vi "Revised-List_Extractor-Mar31.vi"(5 "Input Cluster":T2, 11 "error in (no error)":errorcluster) -> (6 "Output Cluster":T1, 15 "error out":errorcluster)   [LabVIEW 2014]
doc: "This VI extracts and arranges the list of species in an array.\nIn_Arr : Array of species to be arranged\nOut_Arr : Arranged array.\nNote: It does not process list of \"Kinetic Laws\" \n\nDesigned By:\nHB\nhaba@dtu.dk"
panel:
  out "Sp_for_ODE+Names":string[](array[string])
  out "SP_for_ODE_Init_Amnt":string[](array[string])
  out "Sp_for_ODE":string[](array[string])
  out "Ex_Mod_Init_Amnt":string[](array[string])
  out "Rest_Sp_IDs":string[](array[string])
  out "Rest_Sp_Init_Amnt":string[](array[string])
  out "Rest_Sp_IDs+Names":string[](array[string])
  out "Sp_Init_Amount":string[](array[string])
  out "All_Mods":string[](array[string])
  out "Products_Arr":string[](array[string])
  out "Reactants_Arr":string[](array[string])
  out "Ex_Mod_IDs":string[](array[string])
  out "Sp_ID":string[](array[string])
  out "Sp_Name":string[](array[string])
  out "Mod_In_Arr":string[](array[string])
  out "Ex_Mod_IDs+Names":string[](array[string])
  out "strng":string
  out "New mods":string[](array[string])
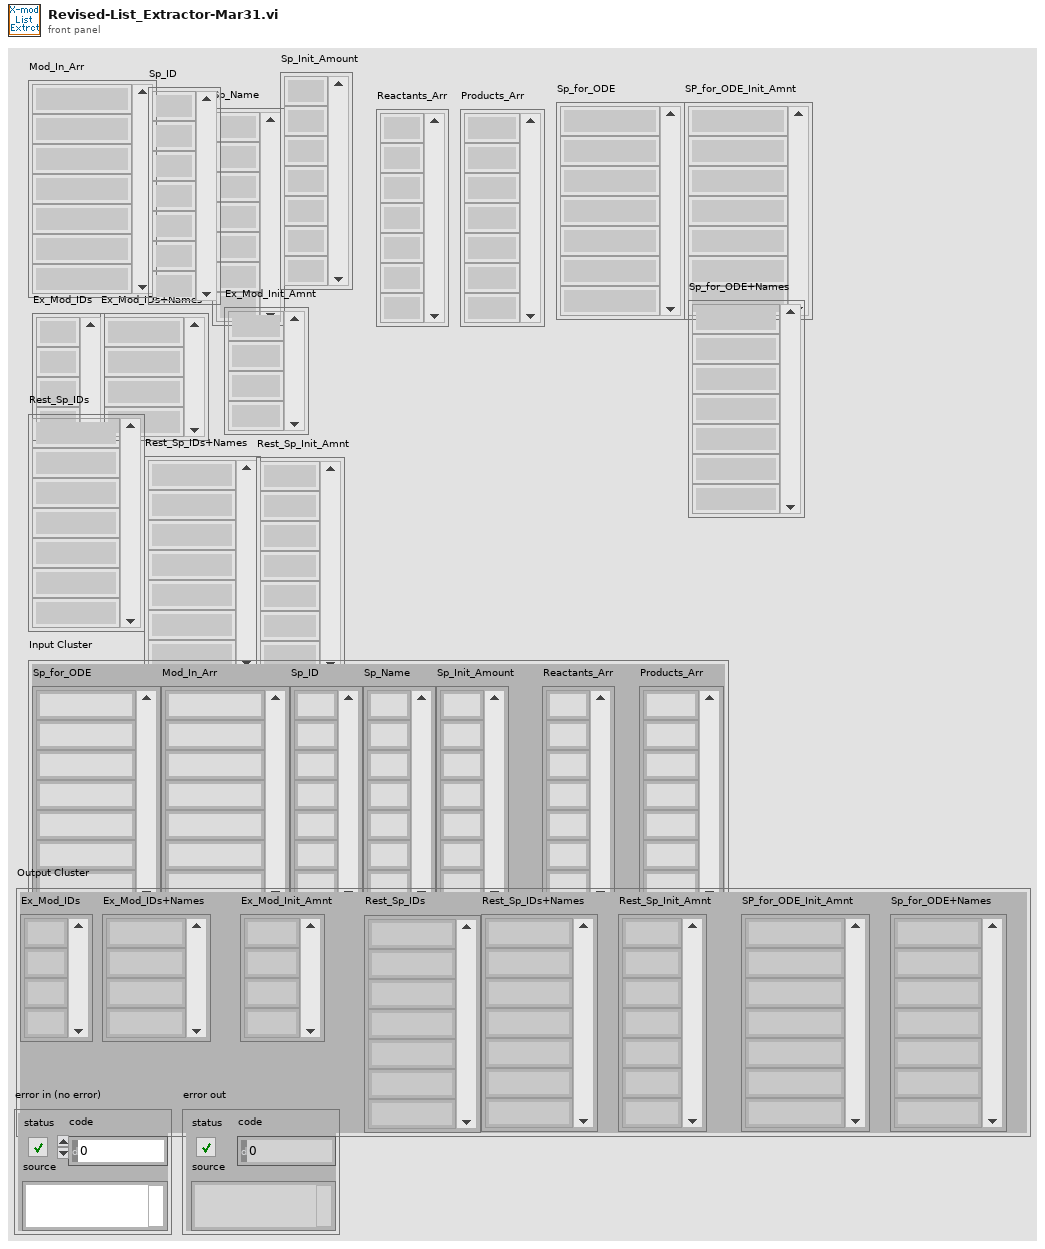
[diagram p1: front panel]
types:
  T1 = cluster{"Ex_Mod_IDs":string[], "Ex_Mod_IDs+Names":string[], "Ex_Mod_Init_Amnt":string[], "Rest_Sp_IDs ":string[], "Rest_Sp_IDs+Names":string[], "Rest_Sp_Init_Amnt":string[], "SP_for_ODE_Init_Amnt":string[], "Sp_for_ODE+Names":string[]}
  T2 = cluster{"Sp_for_ODE":string[], "Mod_In_Arr":string[], "Sp_ID ":string[], "Sp_Name":string[], "Sp_Init_Amount":string[], "Reactants_Arr ":string[], "Products_Arr":string[]}
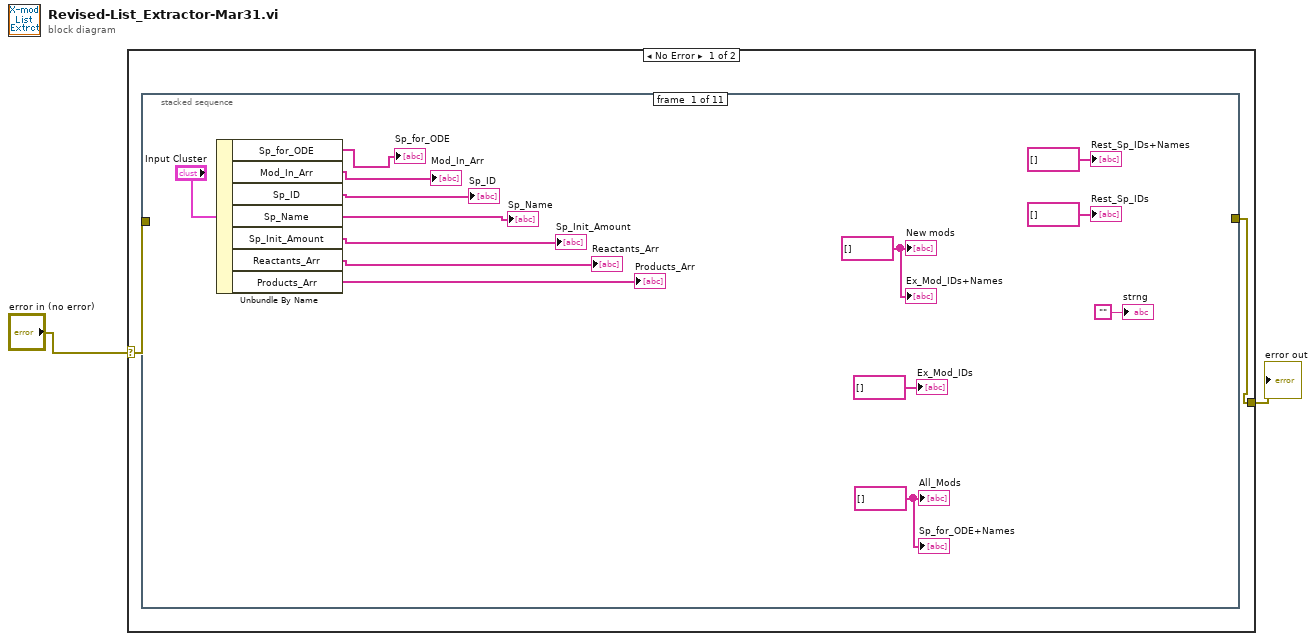
[diagram p0: block diagram]
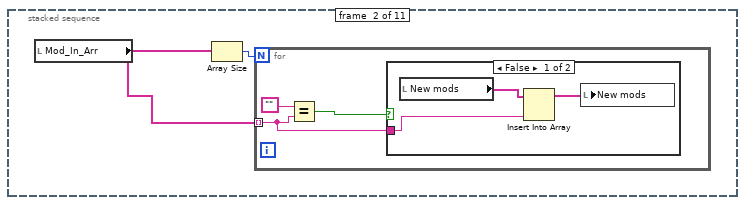
[diagram p2: hidden frame]
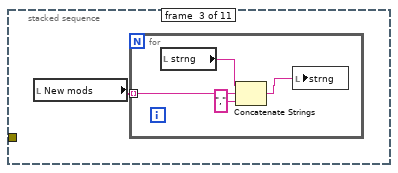
[diagram p4: hidden frame]
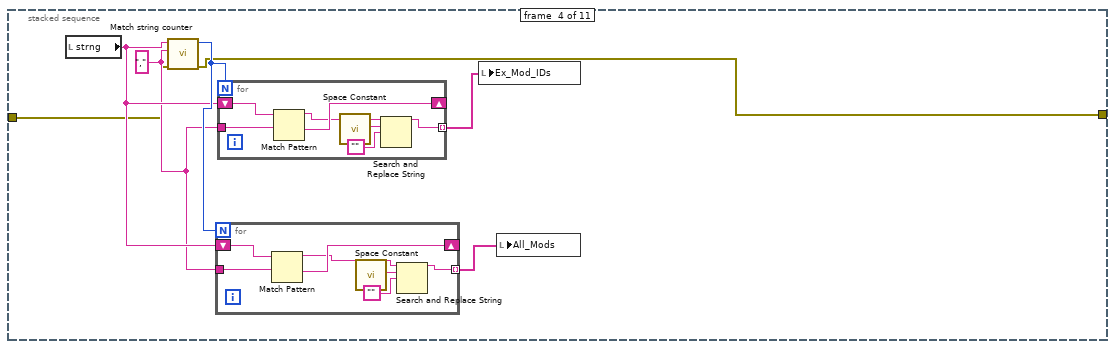
[diagram p5: hidden frame]
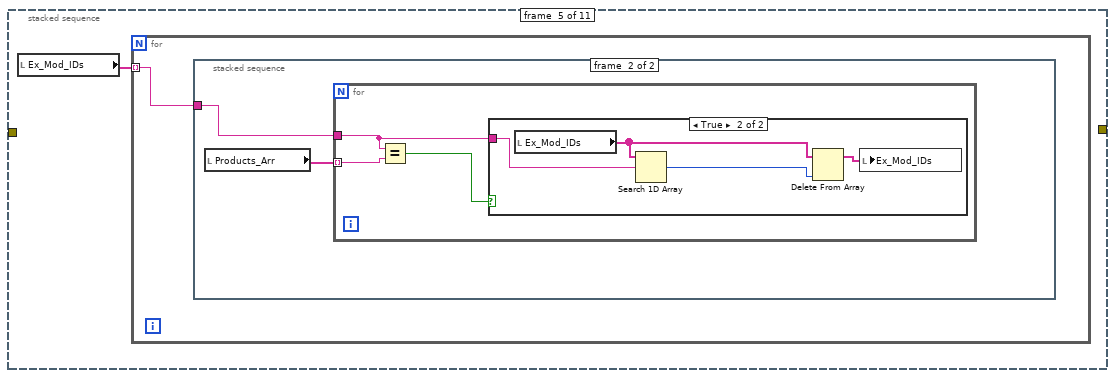
[diagram p6: hidden frame]
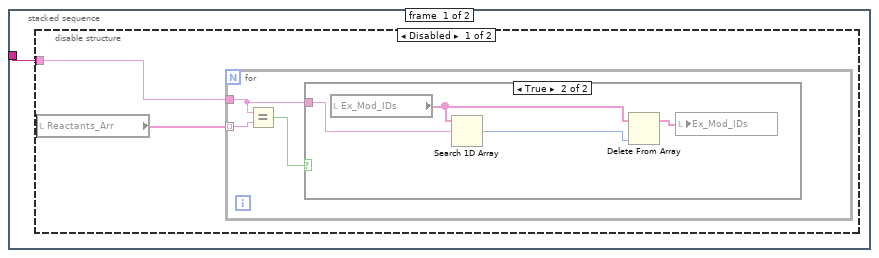
[diagram p7: hidden frame]
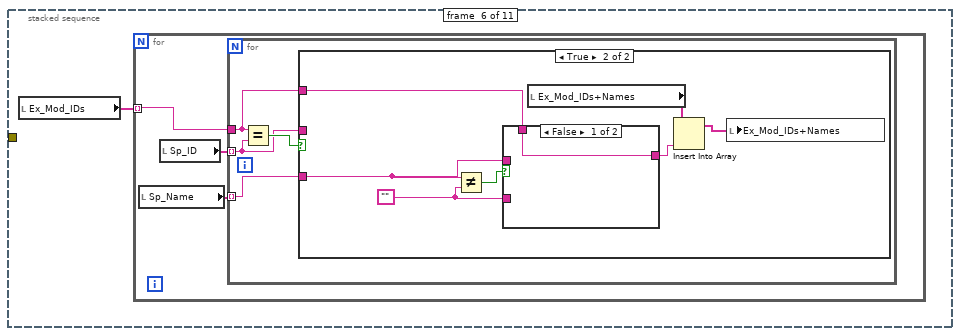
[diagram p11: hidden frame]
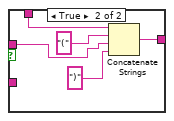
[diagram p13: hidden frame]
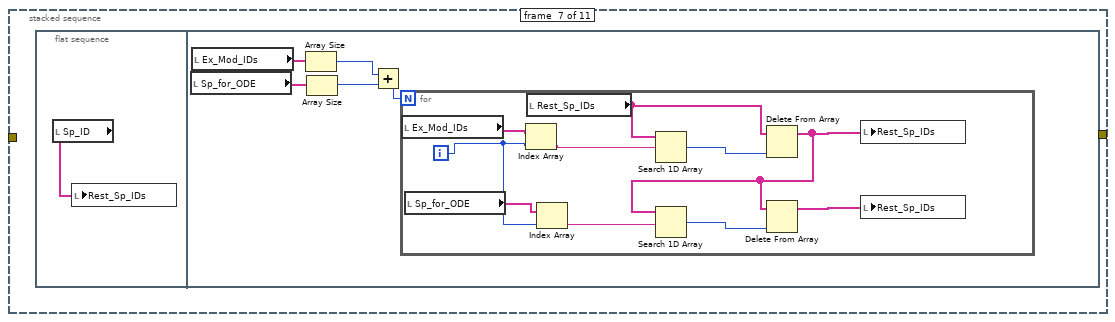
[diagram p14: hidden frame]
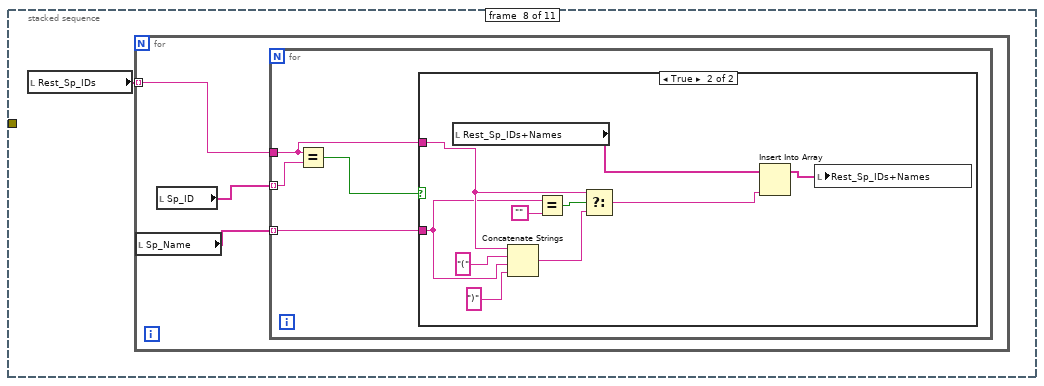
[diagram p15: hidden frame]
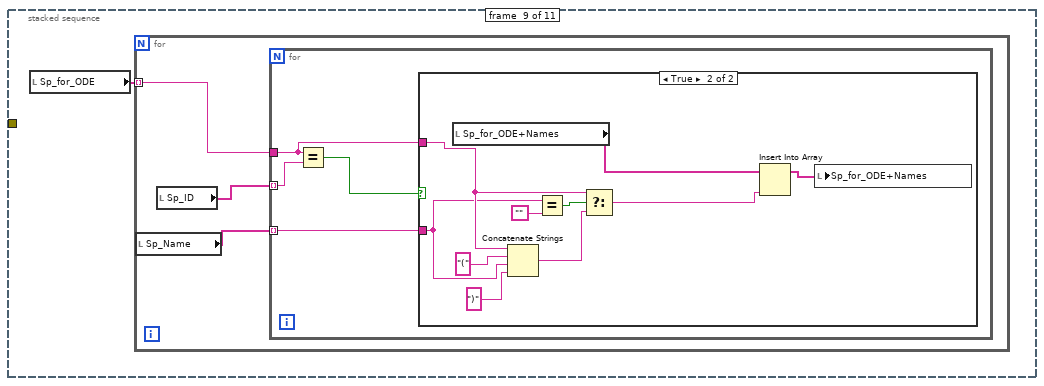
[diagram p17: hidden frame]
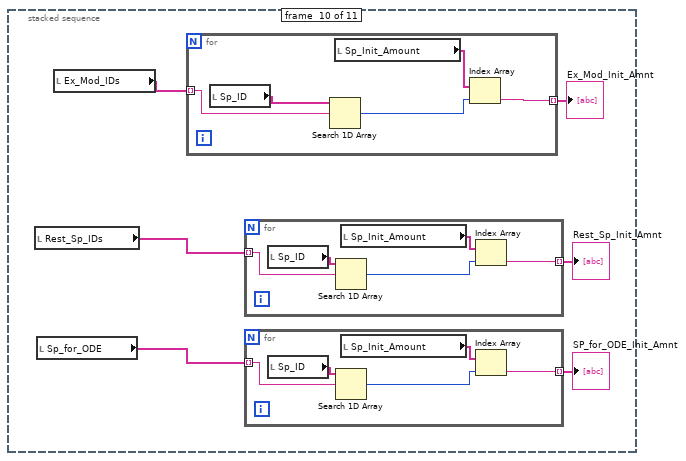
[diagram p19: hidden frame]
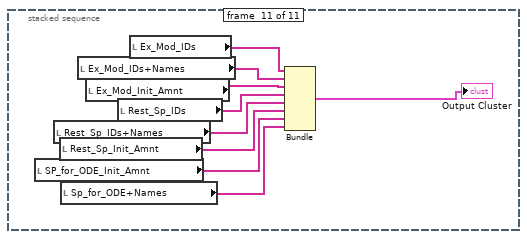
[diagram p20: hidden frame]
diagram:
  n1 = case shown="No Error" "error in (no error)" {
    selector: "error in (no error)" -> [w4 w177]
    tunnel: [w3 w177] -> w1
    frame No Error {
      n2 = stacked-sequence {
        tunnel: w4 -> [_ _ _ w33 _ _ _ _ _ _ _]
        tunnel: [_ _ _ w32 _ _ _ _ _ _ _] -> w3
        frame #0 {
          w13 = string[] [] ("New mods")
          w18 = string[] [] ("New mods")
          n3 = Unbundle By Name("Input Cluster") -> ("Sp_for_ODE"=→"Sp_for_ODE":string[], "Mod_In_Arr"=→"Mod_In_Arr":string[], "Sp_ID"=→"Sp_ID":string[], "Sp_Name"=→"Sp_Name":string[], "Sp_Init_Amount"=→"Sp_Init_Amount":string[], "Reactants_Arr"=→"Reactants_Arr":string[], "Products_Arr"=→"Products_Arr":string[])
          "New mods" <- w18
          "strng" <- ""
          "Ex_Mod_IDs+Names" <- w18
          "Ex_Mod_IDs" <- string[] [] ("New mods")
          "All_Mods" <- w13
          "Rest_Sp_IDs+Names" <- string[] [] ("New mods")
          "Rest_Sp_IDs" <- string[] [] ("New mods")
          "Sp_for_ODE+Names" <- w13
        }
        frame #1 {
          n4 = local read "Mod_In_Arr"() -> (w19:string[])
          n5 = Array Size(array=w19) -> (size(s)=w20:i32)
          n6 = for {
            N: w20 -> [_]
            tunnel: w19 -> [w21] mode=indexing
            n7 = Equal?(x="", y=w21) -> (x = y?=w22:bool)
            n8 = case shown="False" w22 {
              tunnel: w21 -> [w24 _]
              frame False {
                n9 = local read "New mods"() -> (w25:string[])
                n10 = Insert Into Array(array=w25, new element=w24) -> (w26:string[])  [unwired: 1 in]
                n11 = local write "New mods"(w26) -> ()
              }
              frame True {
              }
            }
          }
        }
        frame #2 {
          n12 = local read "New mods"() -> (w27:string[])
          n13 = for {
            tunnel: w27 -> [w30] mode=indexing
            n14 = local read "strng"() -> (w31:string)
            n15 = Concatenate Strings(w31, w30, "," ("string")) -> (w29:string)
            n16 = local write "strng"(w29) -> ()
          }
        }
        frame #3 {
          w34 = "," ("Match String")
          n17 = local read "strng"() -> (w35:string)
          n18 = call "Match string counter.vi"("error in (no error)"=w33, "Match String"=w34, "Input string"=w35) -> ("error out"=w32:errorcluster, "Count"=w36:i32)  [unwired: 7 in]
          n19 = for {
            N: w36 -> [_]
            tunnel: w34 -> [w45]
            tunnel: [w39] -> w37 mode=indexing
            shift-right: [w44] -> _
            shift-left: w35 -> [w43]
            n20 = Match Pattern(string=w43, regular expression=w45) -> (before substring=w40:string, after substring=w44:string)  [unwired: 1 in, 2 out]
            n21 = call <vilib>:"Space Constant.vi"() -> ("String"=w41:string)
            n22 = Search and Replace String(input string=w40, search string=w41, replace string="") -> (result string=w39:string)  [unwired: 5 in, 3 out]
          }
          n23 = for {
            N: w36 -> [_]
            tunnel: w34 -> [w52]
            tunnel: [w48] -> w38 mode=indexing
            shift-right: [w51] -> _
            shift-left: w35 -> [w50]
            n24 = Match Pattern(string=w50, regular expression=w52) -> (before substring=w49:string, after substring=w51:string)  [unwired: 1 in, 2 out]
            n25 = call <vilib>:"Space Constant.vi"() -> ("String"=w47:string)
            n26 = Search and Replace String(input string=w49, search string=w47, replace string="") -> (result string=w48:string)  [unwired: 5 in, 3 out]
          }
          n27 = local write "Ex_Mod_IDs"(w38) -> ()
          n28 = local write "All_Mods"(w37) -> ()
        }
        frame #4 {
          n29 = local read "Ex_Mod_IDs"() -> (w53:string[])
          n30 = for {
            tunnel: w53 -> [w54] mode=indexing
            n31 = stacked-sequence {
              tunnel: w54 -> [w55 w66]
              frame #0 {
                n32 = disable-structure shown="Disabled" {
                  disable-tunnel: w55 -> [w57 _]
                  frame Disabled {
                    n33 = local read "Reactants_Arr"() -> (w56:string[])
                    n34 = for {
                      tunnel: w57 -> [w58]
                      tunnel: w56 -> [w60] mode=indexing
                      n35 = Equal?(x=w58, y=w60) -> (x = y?=w59:bool)
                      n36 = case shown="True" w59 {
                        tunnel: w58 -> [_ w64]
                        frame False {
                        }
                        frame True {
                          n37 = local read "Ex_Mod_IDs"() -> (w62:string[])
                          n38 = Search 1D Array(1D array=w62, element=w64) -> (index of element=w63:i32)  [unwired: 1 in]
                          n39 = Delete From Array(array=w62, index=w63) -> (array with subset deleted=w61:string[])  [unwired: 1 in, 1 out]
                          n40 = local write "Ex_Mod_IDs"(w61) -> ()
                        }
                      }
                    }
                  }
                  frame Enabled {
                  }
                }
              }
              frame #1 {
                n41 = local read "Products_Arr"() -> (w65:string[])
                n42 = for {
                  tunnel: w66 -> [w67]
                  tunnel: w65 -> [w69] mode=indexing
                  n43 = Equal?(x=w67, y=w69) -> (x = y?=w68:bool)
                  n44 = case shown="True" w68 {
                    tunnel: w67 -> [_ w73]
                    frame False {
                    }
                    frame True {
                      n45 = local read "Ex_Mod_IDs"() -> (w71:string[])
                      n46 = Search 1D Array(1D array=w71, element=w73) -> (index of element=w72:i32)  [unwired: 1 in]
                      n47 = Delete From Array(array=w71, index=w72) -> (array with subset deleted=w70:string[])  [unwired: 1 in, 1 out]
                      n48 = local write "Ex_Mod_IDs"(w70) -> ()
                    }
                  }
                }
              }
            }
          }
        }
        frame #5 {
          n49 = local read "Ex_Mod_IDs"() -> (w74:string[])
          n50 = for {
            tunnel: w74 -> [w77] mode=indexing
            n51 = local read "Sp_Name"() -> (w75:string[])
            n52 = local read "Sp_ID"() -> (w76:string[])
            n53 = for {
              tunnel: w75 -> [w80] mode=indexing
              tunnel: w77 -> [w79]
              tunnel: w76 -> [w78] mode=indexing
              n54 = Equal?(x=w79, y=w78) -> (x = y?=w81:bool)
              n55 = case shown="True" w81 {
                tunnel: w80 -> [_ w83]
                tunnel: w79 -> [_ w88]
                tunnel: w78 -> [_ _]
                frame False {
                }
                frame True {
                  w82 = ""
                  n56 = Not Equal?(x=w83, y=w82) -> (x != y?=w84:bool)
                  n57 = case shown="False" w84 {
                    tunnel: w88 -> [w89 w94]
                    tunnel: [w89 w91] -> w85
                    tunnel: w83 -> [_ w90]
                    tunnel: w82 -> [_ _]
                    frame False {
                    }
                    frame True {
                      n58 = Concatenate Strings(w94, "(" ("string"), w90, ")" ("string")) -> (w91:string)
                    }
                  }
                  n59 = local read "Ex_Mod_IDs+Names"() -> (w87:string[])
                  n60 = Insert Into Array(array=w87, new element=w85) -> (w86:string[])  [unwired: 1 in]
                  n61 = local write "Ex_Mod_IDs+Names"(w86) -> ()
                }
              }
            }
          }
        }
        frame #6 {
          n62 = flat-sequence {
            frame #0 {
              n63 = local read "Sp_ID"() -> (w95:string[])
              n64 = local write "Rest_Sp_IDs"(w95) -> ()
            }
            frame #1 {
              n65 = local read "Sp_for_ODE"() -> (w99:string[])
              n66 = local read "Ex_Mod_IDs"() -> (w100:string[])
              n67 = Array Size(array=w100) -> (size(s)=w98:i32)
              n68 = Array Size(array=w99) -> (size(s)=w97:i32)
              n69 = Add(x=w98, y=w97) -> (x+y=w96:i32)
              n70 = for {
                N: w96 -> [_]
                i -> [w104]
                n71 = local read "Ex_Mod_IDs"() -> (w106:string[])
                n72 = local read "Sp_for_ODE"() -> (w103:string[])
                n73 = Index Array(array=w106, index=w104) -> (element=w105:string)
                n74 = local read "Rest_Sp_IDs"() -> (w109:string[])
                n75 = Index Array(array=w103, index=w104) -> (element=w102:string)
                n76 = Search 1D Array(1D array=w109, element=w105) -> (index of element=w110:i32)  [unwired: 1 in]
                n77 = Delete From Array(array=w109, index=w110) -> (array with subset deleted=w101:string[])  [unwired: 1 in, 1 out]
                n78 = Search 1D Array(1D array=w101, element=w102) -> (index of element=w108:i32)  [unwired: 1 in]
                n79 = Delete From Array(array=w101, index=w108) -> (array with subset deleted=w107:string[])  [unwired: 1 in, 1 out]
                n80 = local write "Rest_Sp_IDs"(w101) -> ()
                n81 = local write "Rest_Sp_IDs"(w107) -> ()
              }
            }
          }
        }
        frame #7 {
          n82 = local read "Rest_Sp_IDs"() -> (w111:string[])
          n83 = for {
            tunnel: w111 -> [w113] mode=indexing
            n84 = local read "Sp_Name"() -> (w112:string[])
            n85 = local read "Sp_ID"() -> (w114:string[])
            n86 = for {
              tunnel: w114 -> [w118] mode=indexing
              tunnel: w113 -> [w116]
              tunnel: w112 -> [w115] mode=indexing
              n87 = Equal?(x=w116, y=w118) -> (x = y?=w117:bool)
              n88 = case shown="True" w117 {
                tunnel: w116 -> [_ w124]
                tunnel: w115 -> [_ w122]
                frame False {
                }
                frame True {
                  n89 = local read "Rest_Sp_IDs+Names"() -> (w127:string[])
                  n90 = Concatenate Strings(w124, "(" ("string"), w122, ")" ("string")) -> (w120:string)
                  n91 = Equal?(x=w122, y="") -> (x = y?=w121:bool)
                  n92 = Select(t=w124, s=w121, f=w120) -> (s? t:f=w119:string)
                  n93 = Insert Into Array(array=w127, new element=w119) -> (w128:string[])  [unwired: 1 in]
                  n94 = local write "Rest_Sp_IDs+Names"(w128) -> ()
                }
              }
            }
          }
        }
        frame #8 {
          n95 = local read "Sp_for_ODE"() -> (w129:string[])
          n96 = for {
            tunnel: w129 -> [w131] mode=indexing
            n97 = local read "Sp_Name"() -> (w130:string[])
            n98 = local read "Sp_ID"() -> (w132:string[])
            n99 = for {
              tunnel: w132 -> [w136] mode=indexing
              tunnel: w131 -> [w134]
              tunnel: w130 -> [w133] mode=indexing
              n100 = Equal?(x=w134, y=w136) -> (x = y?=w135:bool)
              n101 = case shown="True" w135 {
                tunnel: w134 -> [_ w142]
                tunnel: w133 -> [_ w140]
                frame False {
                }
                frame True {
                  n102 = local read "Sp_for_ODE+Names"() -> (w145:string[])
                  n103 = Concatenate Strings(w142, "(" ("string"), w140, ")" ("string")) -> (w138:string)
                  n104 = Equal?(x=w140, y="") -> (x = y?=w139:bool)
                  n105 = Select(t=w142, s=w139, f=w138) -> (s? t:f=w137:string)
                  n106 = Insert Into Array(array=w145, new element=w137) -> (w146:string[])  [unwired: 1 in]
                  n107 = local write "Sp_for_ODE+Names"(w146) -> ()
                }
              }
            }
          }
        }
        frame #9 {
          n108 = local read "Rest_Sp_IDs"() -> (w152:string[])
          n109 = local read "Sp_for_ODE"() -> (w148:string[])
          n110 = local read "Ex_Mod_IDs"() -> (w150:string[])
          n111 = for {
            tunnel: w150 -> [w161] mode=indexing
            tunnel: [w158] -> w149 mode=indexing
            n112 = local read "Sp_ID"() -> (w162:string[])
            n113 = Search 1D Array(1D array=w162, element=w161) -> (index of element=w159:i32)  [unwired: 1 in]
            n114 = local read "Sp_Init_Amount"() -> (w160:string[])
            n115 = Index Array(array=w160, index=w159) -> (element=w158:string)
          }
          "Ex_Mod_Init_Amnt" <- w149
          n116 = for {
            tunnel: w152 -> [w166] mode=indexing
            tunnel: [w163] -> w151 mode=indexing
            n117 = local read "Sp_ID"() -> (w167:string[])
            n118 = Search 1D Array(1D array=w167, element=w166) -> (index of element=w164:i32)  [unwired: 1 in]
            n119 = local read "Sp_Init_Amount"() -> (w165:string[])
            n120 = Index Array(array=w165, index=w164) -> (element=w163:string)
          }
          "Rest_Sp_Init_Amnt" <- w151
          n121 = for {
            tunnel: w148 -> [w156] mode=indexing
            tunnel: [w153] -> w147 mode=indexing
            n122 = local read "Sp_ID"() -> (w157:string[])
            n123 = Search 1D Array(1D array=w157, element=w156) -> (index of element=w154:i32)  [unwired: 1 in]
            n124 = local read "Sp_Init_Amount"() -> (w155:string[])
            n125 = Index Array(array=w155, index=w154) -> (element=w153:string)
          }
          "SP_for_ODE_Init_Amnt" <- w147
        }
        frame #10 {
          n126 = local read "SP_for_ODE_Init_Amnt"() -> (w170:string[])
          n127 = local read "Rest_Sp_IDs+Names"() -> (w172:string[])
          n128 = local read "Rest_Sp_Init_Amnt"() -> (w171:string[])
          n129 = local read "Sp_for_ODE+Names"() -> (w169:string[])
          n130 = local read "Ex_Mod_IDs+Names"() -> (w175:string[])
          n131 = local read "Ex_Mod_Init_Amnt"() -> (w174:string[])
          n132 = local read "Rest_Sp_IDs"() -> (w173:string[])
          n133 = local read "Ex_Mod_IDs"() -> (w176:string[])
          n134 = Bundle("Ex_Mod_IDs"=w176, "Ex_Mod_IDs+Names"=w175, "Ex_Mod_Init_Amnt"=w174, "Rest_Sp_IDs"=w173, "Rest_Sp_IDs+Names"=w172, "Rest_Sp_Init_Amnt"=w171, "SP_for_ODE_Init_Amnt"=w170, "Sp_for_ODE+Names"=w169) -> (→"Output Cluster":T1)  [unwired: 1 in]
        }
      }
    }
    frame Error {
    }
  }
  "error out" <- w1
